vi "20211217_00.vi"() -> ()   [LabVIEW 2019]
panel:
  out "Console Log":string
  out "Light":bool
  in  "Button":bool
  in  "TUR.LIGHT":bool
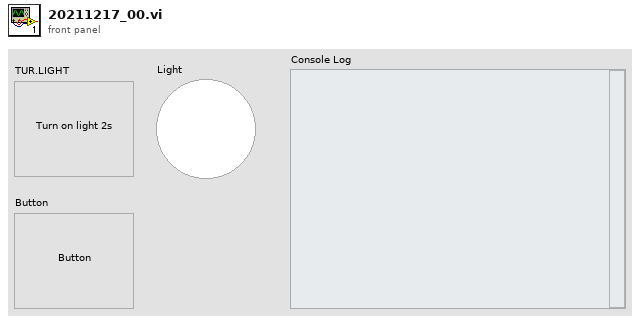
[diagram p1: front panel]
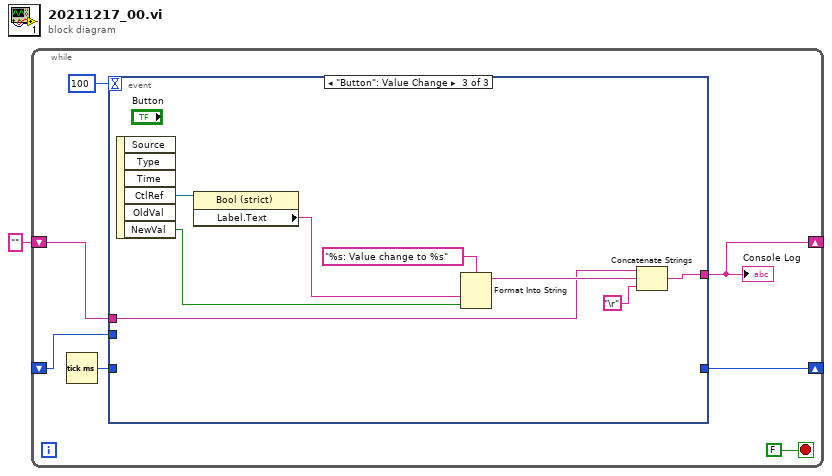
[diagram p0: block diagram]
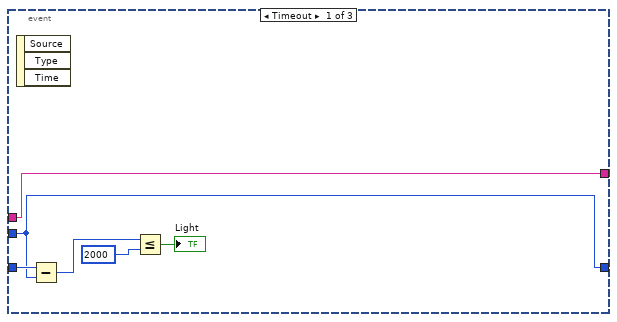
[diagram p2: hidden frame]
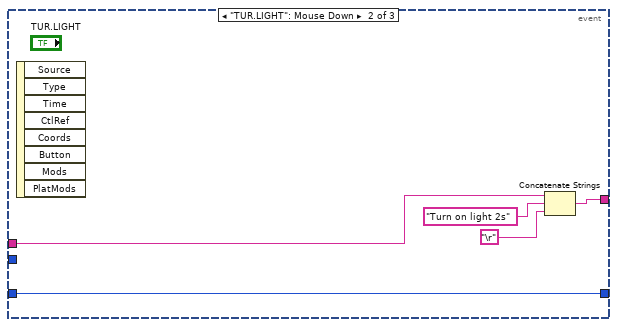
[diagram p3: hidden frame]
diagram:
  n1 = while {
    shift-right: [w6] -> _
    shift-left: _ -> [w4]
    shift-right: [w3] -> _
    shift-left: "" -> [w2]
    stop <- FALSE stop-if-true
    n2 = Tick Count (ms)() -> (millisecond timer value=w5:u32)
    n3 = event shown="[2] \"Button\": Value Change" {
      selector: _ -> [_ _ _]
      dyn-events: _ -> [_ _ _]
      timeout: 100 -> [_ _ _]
      tunnel: [w10 w19 _] -> w6
      tunnel: w5 -> [w14 w19 _]
      tunnel: w4 -> [w10 _ _]
      tunnel: [w9 w18 w23] -> w3
      tunnel: w2 -> [w9 w17 w22]
      event Timeout {
        n4 = event-data() -> ()  [unwired: 1 in, 3 out]
        n5 = Subtract(x=w14, y=w10) -> (x-y=w13:u32)
        n6 = Less Or Equal?(x=w13, y=u32 2000) -> (x <= y?=→"Light":bool)
      }
      event "TUR.LIGHT": Mouse Down {
        n7 = event-data() -> ()  [unwired: 1 in, 8 out]
        n8 = Concatenate Strings(w17, "Turn on light 2s" ("string"), "\r") -> (w18:string)
      }
      event "Button": Value Change {
        n9 = event-data() -> ("CtlRef"=w27:refnum<vi>, "NewVal"=w25:bool)  [unwired: 1 in, 4 out]
        n10 = property class="Bool (strict)"(reference=w27) -> ("Label.Text"=w26:string)  [unwired: 1 in, 2 out]
        n11 = Format Into String(format string="%s: Value change to %s" ("initial string"), w26, w25) -> (resulting string=w24:string)  [unwired: 2 in, 1 out]
        n12 = Concatenate Strings(w22, w24, "\r") -> (w23:string)
      }
    }
    "Console Log" <- w3
  }
